vi "rising edge toggle.vi"(1 "toggle 2":dbl, 2 "Control":bool, 3 "toggle 1":dbl) -> (0 "output":dbl)   [LabVIEW 2012]
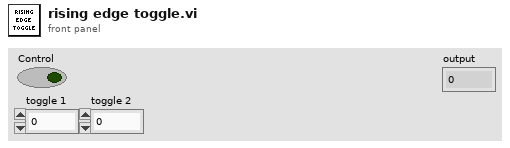
[diagram p1: front panel]
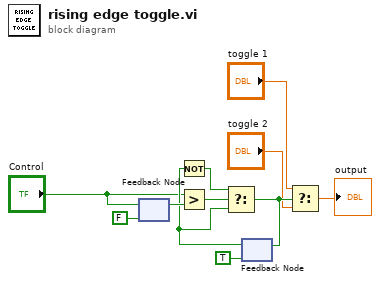
[diagram p0: block diagram]
diagram:
  n1 = feedback #1(FALSE ("L Drive Button 5")) -> (w11:bool)
  n2 = feedback-in #1("Control") -> ()
  n3 = Greater?(x="Control", y=w11) -> (0:w9:bool)
  n4 = feedback #2(TRUE) -> (w7:bool)
  n5 = Not(x=w7) -> (.not. x?=w8:bool)
  n6 = Select(t=w8, s=w9, f=w7) -> (s? t:f=w4:bool)
  n7 = feedback-in #2(w4) -> ()
  n8 = Select(t="toggle 1", s=w4, f="toggle 2") -> (s? t:f=→"output":dbl)
